vi "DOE Dryer PreCondition Stabilize Temperatures.vi"(7 "Temps":dbl[](array[numeric]), 8 "Error In":errorcluster, 10 "15 Min":dbl=600.0, 11 "Timer":dbl) -> (0 "Error Out":errorcluster, 2 "15 min Up":bool, 3 "Temp stable":bool)   [LabVIEW 2016]
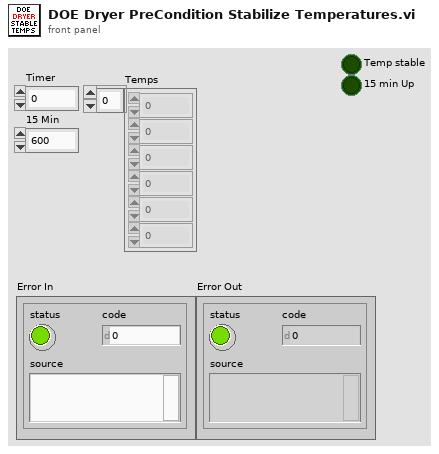
[diagram p1: front panel]
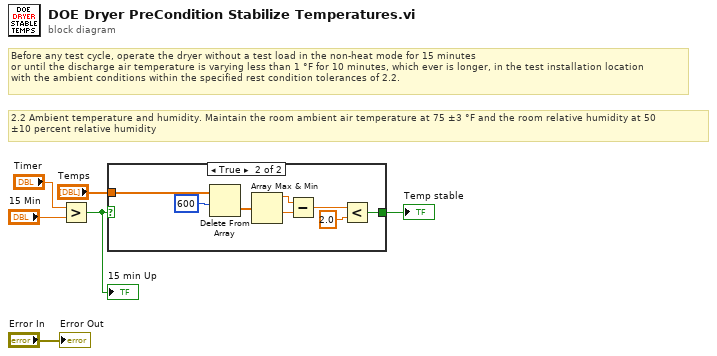
[diagram p0: block diagram]
diagram:
  # "2.2 Ambient temperature and humidity. Maintain the room ambient air temperature at 75 ±3 °F and the room relative humidity at 50\n±10 percent relative humidity"
  # "Before any test cycle, operate the dryer without a test load in the non-heat mode for 15 minutes\nor until the discharge air temperature is varying less than 1 °F for 10 minutes, which ever is longer, in the test installation location\nwith the ambient conditions within the specified rest condition tolerances of 2.2."
  n1 = Greater?(x="Timer", y="15 Min") -> (0:w5:bool)
  "15 min Up" <- w5
  n2 = case shown="True" w5 {
    selector: w5 -> [w7 _]
    tunnel: [w7 w8] -> w6
    tunnel: "Temps" -> [_ w15]
    frame False {
    }
    frame True {
      n3 = Delete From Array(array=w15, length=600) -> (deleted portion=w13:dbl[])  [unwired: 1 in, 1 out]
      n4 = Array Max & Min(array=w13) -> (max value=w12:dbl, min value=w11:dbl)  [unwired: 2 out]
      n5 = Subtract(x=w12, y=w11) -> (x-y=w10:dbl)
      n6 = Less?(x=w10, y=2.0) -> (x < y?=w8:bool)
    }
  }
  "Temp stable" <- w6
  "Error Out" <- "Error In"
